vi "ImageManipulating.vi"() -> ()   [LabVIEW 2021]
panel:
  in  "gamma":dbl(knob) scale=0.0..1.0
  in  "Salida":path
  out "Waveform Graph 2":dbl[][](graph)
  out "Waveform Graph":dbl[][](graph)
  in  "sig":dbl(knob) scale=0.0..255.0
  in  "u":dbl(knob) scale=0.0..255.0
  in  "P":dbl(knob) scale=0.0..255.0
  in  "c":dbl(knob) scale=0.0..255.0
  out "XY Graph":cluster{i32[], dbl[]}(graph)
  in  "Enum":T1(ring)
  out "new picture":picture
  in  "Path":path
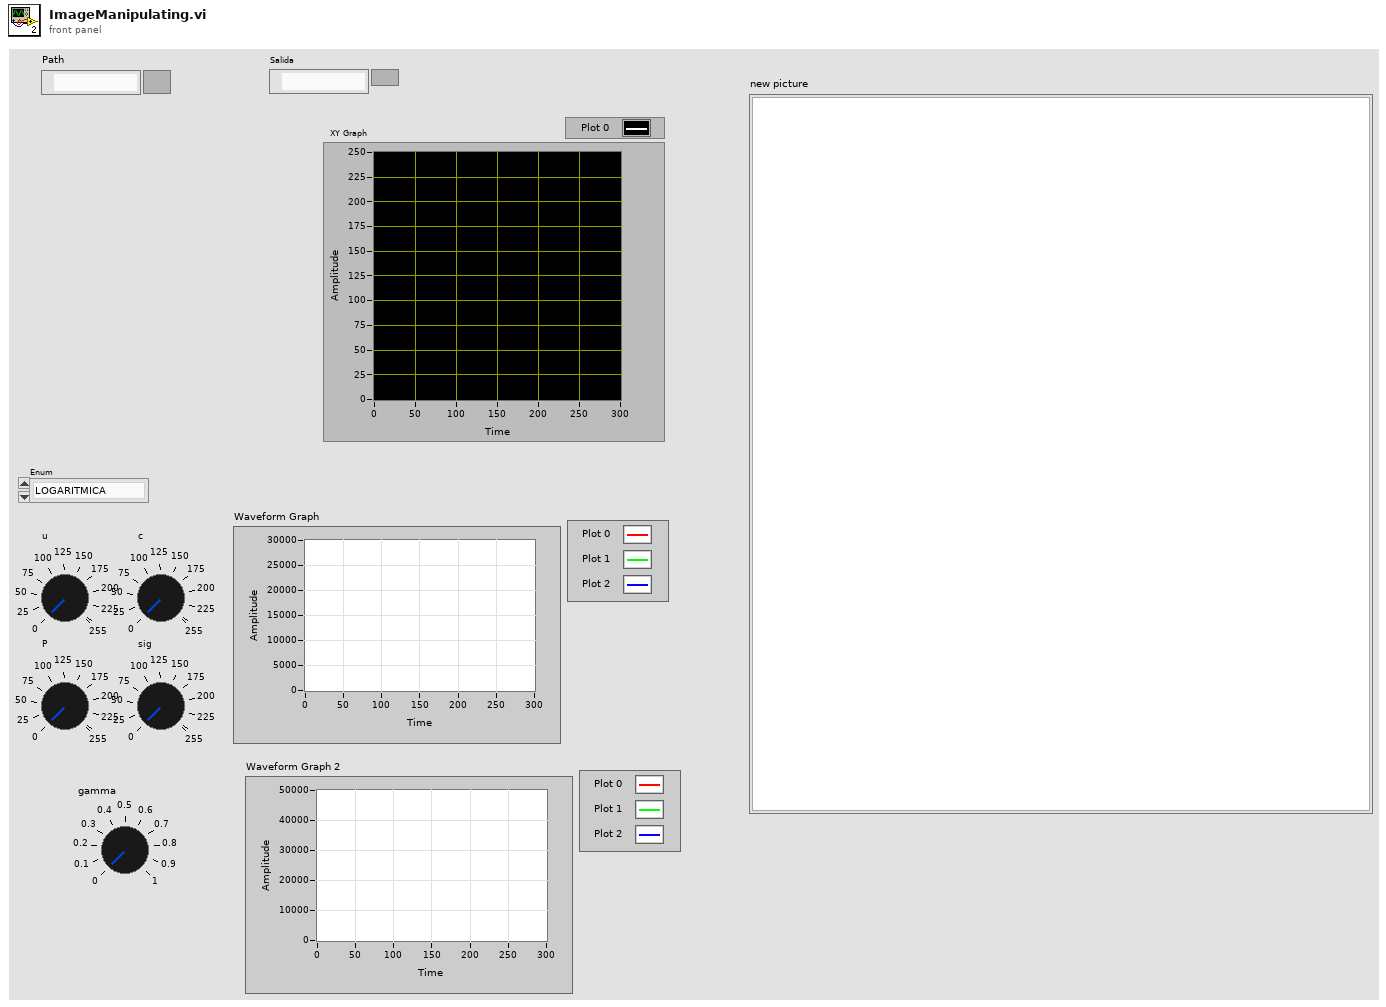
[diagram p1: front panel]
types:
  T1 = enum16{"LOGARITMICA", "GAUSSIANA", "POTENCIA INVERTIDA", "POTENCIA", "RAIZ", "CUADRADA", "EXPONENCIAL", "LINEAL", "Gamma"}
  T2 = typedef "imagedata.ctl" = cluster{"image type":i32, "image depth":i32, "image":u8[], "mask":u8[], "colors":u32[], "Rectangle":cluster{"left":i16, "top":i16, "right":i16, "bottom":i16}}
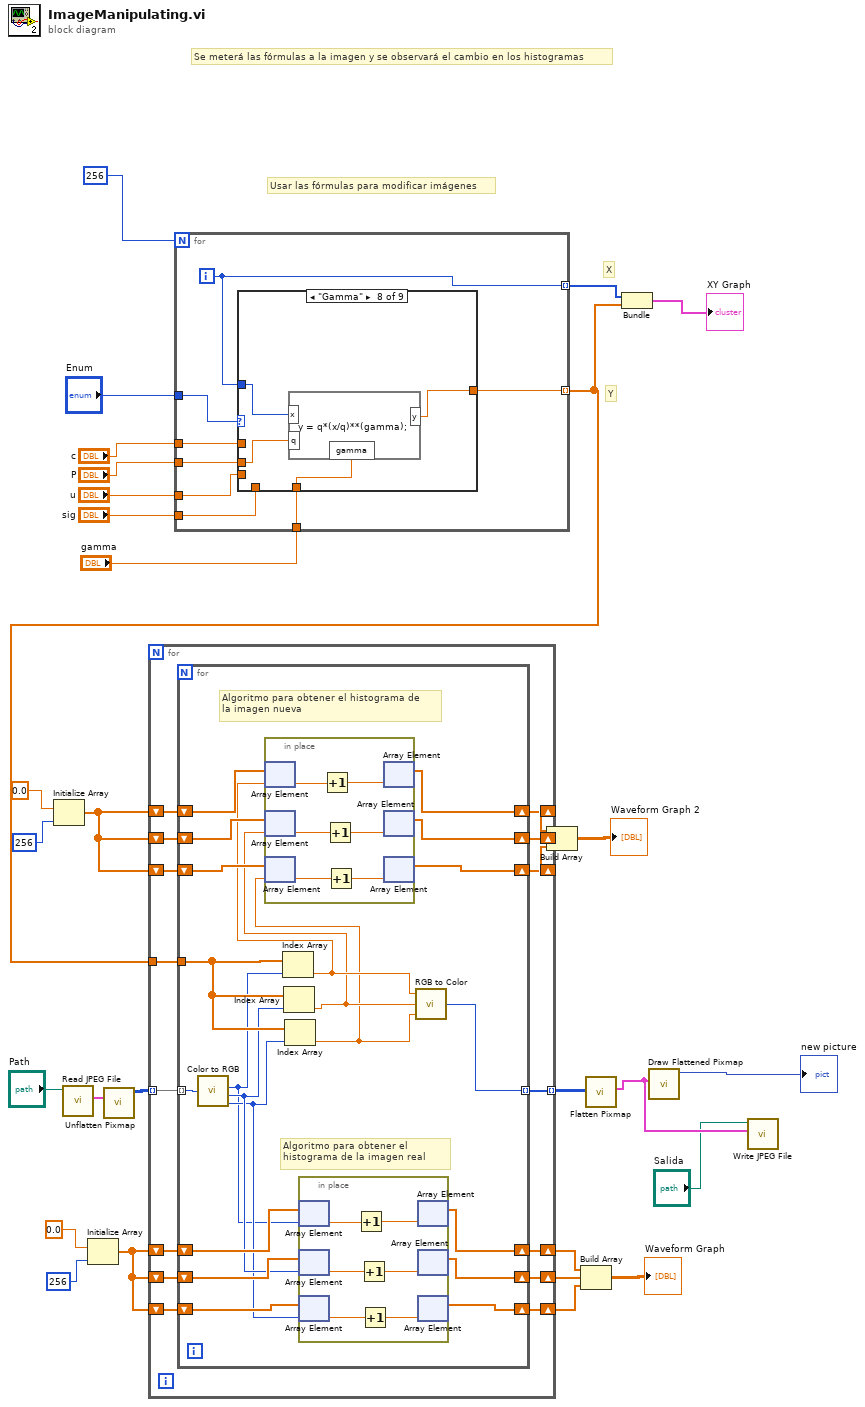
[diagram p0: block diagram]
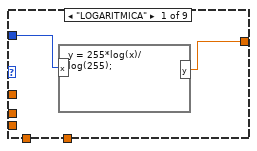
[diagram p2: hidden frame]
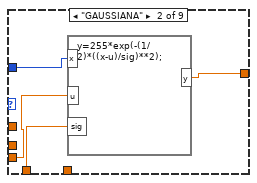
[diagram p3: hidden frame]
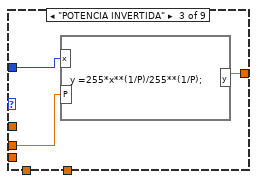
[diagram p4: hidden frame]
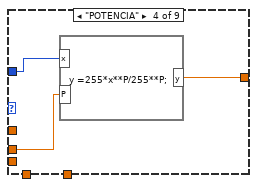
[diagram p5: hidden frame]
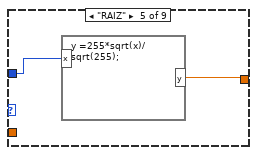
[diagram p6: hidden frame]
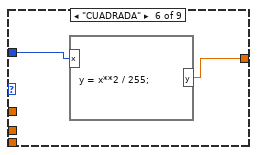
[diagram p7: hidden frame]
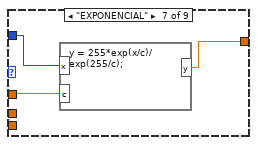
[diagram p8: hidden frame]
diagram:
  # "Usar las fórmulas para modificar imágenes"
  # "Se meterá las fórmulas a la imagen y se observará el cambio en los histogramas"
  # "Y"
  # "X"
  n1 = Initialize Array(0.0 ("element"), 256 ("dimension size")) -> (w10:dbl[])
  n2 = call <vilib>:"Read JPEG File.vi"("path to JPEG file"="Path") -> ("image data"=w30:T2)  [unwired: 8 in, 2 out]
  n3 = Initialize Array(0.0 ("element"), 256 ("dimension size")) -> (w20:dbl[])
  n4 = call <vilib>:"Unflatten Pixmap.vi"("image data"=w30) -> ("24-bit pixmap"=w28:u32[][])  [unwired: 4 in, 6 out]
  n5 = for {
    N: 256 -> [_]
    tunnel: [w38] -> w24 mode=indexing
    tunnel: "Enum" -> [w39]
    tunnel: [w37] -> w15 mode=indexing
    tunnel: "c" -> [w36]
    tunnel: "P" -> [w35]
    tunnel: "u" -> [w34]
    tunnel: "sig" -> [w33]
    tunnel: "gamma" -> [w32]
    i -> [w38]
    n6 = case shown="\"Gamma\"" w39 {
      tunnel: w38 -> [w41 w43 w48 w50 w53 w54 w58 w62 w63]
      tunnel: [w40 w42 w47 w49 w52 w55 w57 w61 w63] -> w37
      tunnel: w36 -> [_ _ _ _ _ _ w56 _ _]
      tunnel: w35 -> [_ _ w46 w51 _ _ _ w59 _]
      tunnel: w34 -> [_ w44 _ _ _ _ _ _ _]
      tunnel: w33 -> [_ w45 _ _ _ _ _ _ _]
      tunnel: w32 -> [_ _ _ _ _ _ _ w60 _]
      frame "LOGARITMICA" {
        n7 = formula code="y = 255*log(x)/log(255);"("x"=w41) -> ("y"=w40:dbl)
      }
      frame "GAUSSIANA" {
        n8 = formula code="y=255*exp(-(1/2)*((x-u)/sig)**2);"("x"=w43, "u"=w44, "sig"=w45) -> ("y"=w42:dbl)
      }
      frame "POTENCIA INVERTIDA" {
        n9 = formula code="y =255*x**(1/P)/255**(1/P);"("x"=w48, "P"=w46) -> ("y"=w47:dbl)
      }
      frame "POTENCIA" {
        n10 = formula code="y =255*x**P/255**P;"("x"=w50, "P"=w51) -> ("y"=w49:dbl)
      }
      frame "RAIZ" {
        n11 = formula code="y =255*sqrt(x)/sqrt(255);"("x"=w53) -> ("y"=w52:dbl)
      }
      frame "CUADRADA" {
        n12 = formula code="y = x**2 / 255;"("x"=w54) -> ("y"=w55:dbl)
      }
      frame "EXPONENCIAL" {
        n13 = formula code="y = 255*exp(x/c)/exp(255/c);"("x"=w58, "c"=w56) -> ("y"=w57:dbl)
      }
      frame "Gamma" {
        n14 = formula code="y = q*(x/q)**(gamma);"("x"=w62, "gamma"=w60, "q"=w59) -> ("y"=w61:dbl)
      }
      frame "LINEAL", Default {
      }
    }
  }
  n15 = for {
    tunnel: w28 -> [w78] mode=indexing
    tunnel: [w77] -> w27 mode=indexing
    shift-right: [w73] -> w19
    shift-left: w20 -> [w76]
    shift-right: [w72] -> w18
    shift-left: w20 -> [w75]
    shift-right: [w71] -> w17
    shift-left: w20 -> [w74]
    tunnel: w15 -> [w70]
    shift-right: [w67] -> w11
    shift-left: w10 -> [w64]
    shift-right: [w68] -> w12
    shift-left: w10 -> [w65]
    shift-right: [w69] -> w13
    shift-left: w10 -> [w66]
    n16 = for {
      tunnel: w78 -> [w98] mode=indexing
      tunnel: [w99] -> w77 mode=indexing
      shift-right: [w96] -> w73
      shift-left: w76 -> [w97]
      shift-right: [w93] -> w72
      shift-left: w75 -> [w95]
      shift-right: [w92] -> w71
      shift-left: w74 -> [w94]
      tunnel: w70 -> [w91]
      shift-right: [w83] -> w67
      shift-left: w64 -> [w82]
      shift-right: [w86] -> w68
      shift-left: w65 -> [w84]
      shift-right: [w87] -> w69
      shift-left: w66 -> [w85]
      # "Algoritmo para obtener el histograma de \nla imagen nueva"
      # "Algoritmo para obtener el histograma de la imagen real"
      n17 = call <vilib>:"Color to RGB.vi"("Color"=w98) -> ("R"=w88:u8, "G"=w90:u8, "B"=w89:u8)  [unwired: 1 out]
      n18 = Index Array(array=w91, index=w88) -> (element=w81:dbl)
      n19 = Index Array(array=w91, index=w90) -> (element=w80:dbl)
      n20 = Index Array(array=w91, index=w89) -> (element=w79:dbl)
      n21 = in-place {
        n22 = in-place-array #1(w82, w81) -> (w105:dbl)
        n23 = in-place-array #2(w84, w80) -> (w102:dbl)
        n24 = in-place-array #3(w85, w79) -> (w103:dbl)
        n25 = Increment(x=w105) -> (x+1=w104:dbl)
        n26 = Increment(x=w102) -> (x+1=w101:dbl)
        n27 = Increment(x=w103) -> (x+1=w100:dbl)
        n28 = in-place-array #1(w104) -> (w83:dbl[])  [unwired: 1 out]
        n29 = in-place-array #2(w101) -> (w86:dbl[])  [unwired: 1 out]
        n30 = in-place-array #3(w100) -> (w87:dbl[])  [unwired: 1 out]
      }
      n31 = in-place {
        n32 = in-place-array #4(w97, w88) -> (w111:dbl)
        n33 = in-place-array #5(w95, w90) -> (w108:dbl)
        n34 = in-place-array #6(w94, w89) -> (w109:dbl)
        n35 = Increment(x=w111) -> (x+1=w110:dbl)
        n36 = Increment(x=w108) -> (x+1=w107:dbl)
        n37 = Increment(x=w109) -> (x+1=w106:dbl)
        n38 = in-place-array #4(w110) -> (w96:dbl[])  [unwired: 1 out]
        n39 = in-place-array #5(w107) -> (w93:dbl[])  [unwired: 1 out]
        n40 = in-place-array #6(w106) -> (w92:dbl[])  [unwired: 1 out]
      }
      n41 = call <vilib>:"RGB to Color.vi"("B"=w79, "G"=w80, "R"=w81) -> ("Color"=w99:u32)
    }
  }
  n42 = Build Array(w11, w12, w13) -> (→"Waveform Graph 2":dbl[][])
  n43 = Build Array(w19, w18, w17) -> (→"Waveform Graph":dbl[][])
  n44 = call <vilib>:"Flatten Pixmap.vi"("24-bit pixmap"=w27) -> ("image data"=w3:T2)  [unwired: 10 in]
  n45 = Bundle(w24, w15) -> (→"XY Graph":cluster{i32[], dbl[]})  [unwired: 1 in]
  n46 = call <vilib>:"Draw Flattened Pixmap.vi"("image data"=w3) -> ("new picture"=→"new picture":picture)  [unwired: 8 in]
  n47 = call <vilib>:"Write JPEG File.vi"("image data"=w3, "path to JPEG file"="Salida") -> ()  [unwired: 8 in, 2 out]
